vi "State_Machine.vi"(8 "error in (no error)":errorcluster caption="entrée d'erreur (pas d'erreur)", 11 "Get_Voltage en entrée":refnum<class "P2056_Wait_Start.lvclass">) -> (0 "error out":errorcluster caption="sortie d'erreur", 2 "Json_String":string, 3 "Get_Voltage en sortie":refnum<class "P2056_Wait_Start.lvclass">)   [LabVIEW 2020, in "Library Test.lvlib" / "P2056_Wait_Start.lvclass"]
uses:
  P2056_Wait_Start.lvclass
  C:/Users/ngarcin/OneDrive - Altyor/Standard TB/Class/Test/Test (Default)/Test (Default).lvclass
  Commun VI/TypeDef/Commande UART/Parametre UART.ctl
  UART/UART (Default)/Class UART (Default).lvclass
  JSON API/JSON Value/Set from JSON string.vi
  a224be2c-9436-4493-a39a-966efb3049a6.vi
  Instrument/Instrument (Default)/Class Instrument (Default).lvclass
  JSON API/JSON Value/JSON Value.lvclass
  P2056_Wait_Start.lvclass/P2056_Wait_Start.ctl
  JSON API/Variant JSON/Variant JSON.lvlib
  JSON API/Get Polymorphic/JSON GetSet.lvlib
  Commun VI/Library Commun.lvlib
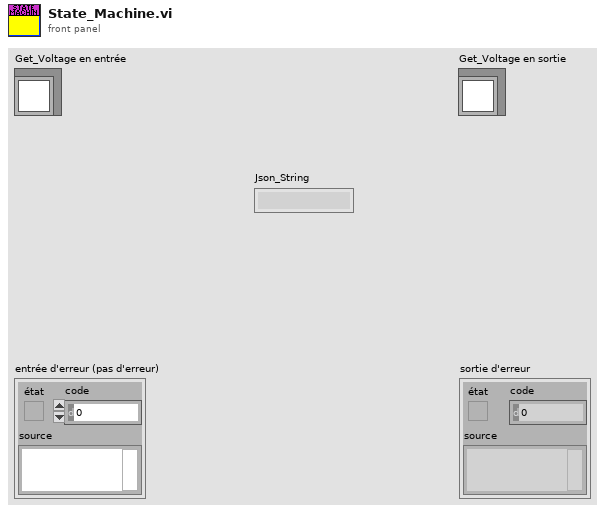
[diagram p1: front panel]
types:
  T1 = typedef "Parametre UART.ctl" = cluster{"Address Device":refnum<visa-resource-name>, "Baud Rate":u32, "Data Bit":u16, "stop bits (10: 1 bit)":u16, "parity (0:none)":enum16{"None", "Odd", "Even", "Mark", "Space"}, "flow control (0:none)":u16, "termination char ":u8, "Enable Termination":bool, "Nb Octet to Read":u16, "Class UART":refnum<class "Class UART (Default).lvclass">}
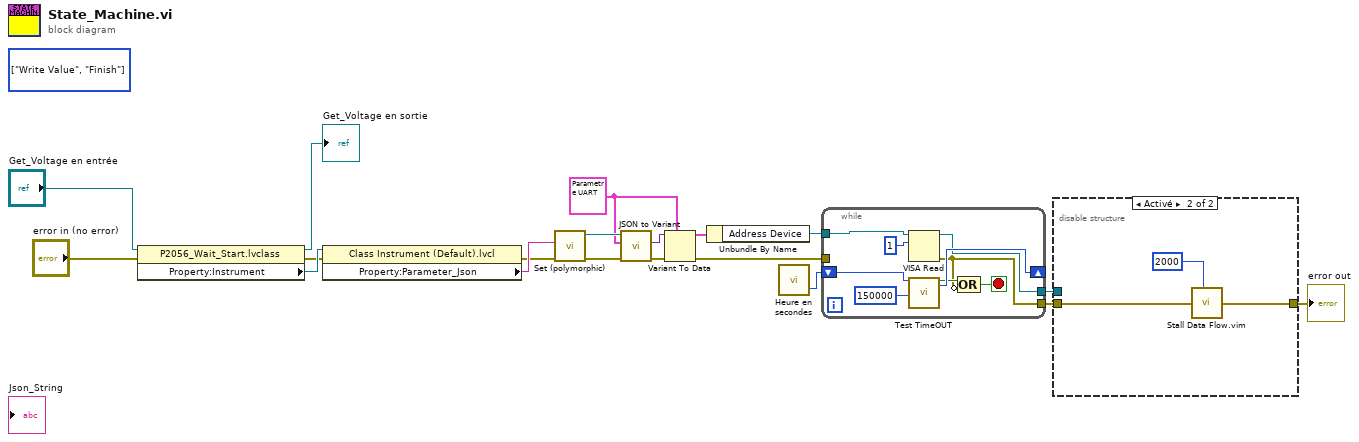
[diagram p0: block diagram]
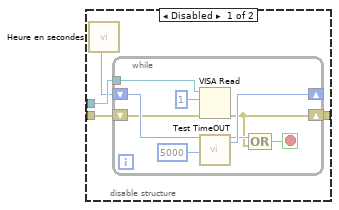
[diagram p2: hidden frame]
diagram:
  w10 = T1 {"Address Device"="", "Baud Rate"=0, "Data Bit"=0, "stop bits (10: 1 bit)"=0, "parity (0:none)"=enum."None", "flow control (0:none)"=0, "termination char "=0, "Enable Termination"=FALSE, "Nb Octet to Read"=0, "Class UART"=refnum} ("Parameter")
  (unwired) enum16{"Init", "Write Value", "Finish"}[] [enum."Write Value", enum."Finish"] items=["Init", "Write Value", "Finish"]
  n1 = property class="P2056_Wait_Start.lvclass"(reference="Get_Voltage en entrée", error in="error in (no error)") -> (reference out=→"Get_Voltage en sortie":refnum<class "P2056_Wait_Start.lvclass">, error out=w7:errorcluster, "Property:Instrument"=w19:refnum<class "Class Instrument (Default).lvclass">)
  n2 = property class="Class Instrument (Default).lvcl"(reference=w19, error in=w7) -> (error out=w6:errorcluster, "Property:Parameter_Json"=w11:string)  [unwired: 1 out]
  n3 = call-poly "Set (polymorphic).vi"("error in (no error)"=w6, "JSON stream"=w11) -> ("error out"=w13:errorcluster, "JSON Value out"=w15:refnum<class "JSON Value.lvclass">)  [unwired: 7 in, 1 out]
  n4 = call "JSON to Variant.vi"("error in (no error)"=w13, "Variant (Data Type)"=w10, "JSON Value"=w15) -> ("error out"=w14:errorcluster, "Variant out"=w12:variant)  [unwired: 7 in]
  n5 = Variant To Data(error in=w14, type=w10, Variant=w12) -> (data=w9:T1, error out=w4:errorcluster)
  n6 = Unbundle By Name(w9) -> ("Address Device"=w8:refnum<visa-resource-name>)
  n7 = call "Heure en secondes.vi"() -> ("Heure en milisecondes"=w5:u32)  [unwired: 2 in, 1 out]
  n8 = while {
    tunnel: w8 -> [w27]
    shift-right: [w25] -> _
    shift-left: w5 -> [w26]
    tunnel: w4 -> [_]
    tunnel: [w22] -> w3
    tunnel: [w20] -> w1
    stop <- w21 stop-if-true
    n9 = VISA Read(VISA resource name=w27, byte count=u32 1 ("nombre d'octets")) -> (VISA resource name out=w20:refnum<visa-resource-name>, error out=w22:errorcluster)  [unwired: 1 in, 2 out]
    n10 = call "Test TimeOUT.vi"("OLD Time"=w26, "TimeOut ms"=u32 150000) -> ("Timeout ?"=w23:bool, "NEW Time"=w25:u32)  [unwired: 13 in, 3 out]
    n11 = Compound Arithmetic op=OR ("Opérateur arithmétique")(w23, invert w22) -> (w21:bool)
  }
  n12 = disable-structure shown="Activé" {
    disable-tunnel: w3 -> [w32 w44]
    disable-tunnel: [w31 w43] -> w2
    disable-tunnel: w1 -> [w30 _]
    frame Disabled {
      n13 = call "Heure en secondes.vi"() -> ("Heure en milisecondes"=w29:u32)  [unwired: 2 in, 1 out]
      n14 = while {
        tunnel: w30 -> [w40]
        shift-right: [w38] -> _
        shift-left: w29 -> [w39]
        shift-right: [w35] -> w31
        shift-left: w32 -> [w33]
        stop <- w34 stop-if-true
        n15 = VISA Read(VISA resource name=w40, byte count=u32 1 ("nombre d'octets"), error in (no error)=w33) -> (error out=w35:errorcluster)  [unwired: 3 out]
        n16 = call "Test TimeOUT.vi"("OLD Time"=w39, "TimeOut ms"=u32 5000) -> ("Timeout ?"=w36:bool, "NEW Time"=w38:u32)  [unwired: 13 in, 3 out]
        n17 = Compound Arithmetic op=OR ("Opérateur arithmétique")(w36, w35) -> (w34:bool)
      }
    }
    frame Enabled {
      n18 = call "Stall Data Flow.vim"("value in"=w44, "milliseconds to wait"=u32 2000) -> ("value out"=w43:errorcluster)  [unwired: 1 out]
    }
  }
  "error out" <- w2
